vi "Radar_Wireless_2Radars.vi"(0 "VISA resource name":refnum<visa-resource-name>="COM1", 1 "baud rate":u32=9600, 4 "data bits":u16=8 min=5 max=8 step=1, 5 "parity":u16(ring) items=["None", "Odd", "Even", "Mark", "Space"], 7 "stop bits":u16(ring)=10 items=["1.0"=10, "1.5"=15, "2.0"=20], 9 "XON Character":u8=17 format="%.0x", 14 "XOFF Character":u8=19 format="%.0x", 15 "timeout (ms)":u32=10000, 21 "End read on termination character?":bool=TRUE, 24 "termination char\n(0xA = '\\n' = LF)":u8=10 format="%.0x", 25 "Input\nbuffer size":u32=4096) -> ()   [LabVIEW 2010]
doc: "The Advanced Serial Read and Write example performs a Serial Port Read, a Serial Port Write, or a combination of these actions while setting some advanced serial features like buffer size, termination characters, and XON/XOFF flow control. The user selects the actions (read or write) on the front panel. If both are selected, the VI will write the data first, read the data and then close the VISA session that is opened to the port. \n\nThe parameters set for the serial port must match the parameters of the connected instrument or device. In this example, the bytes to read parameter specifies the number of bytes that the serial port reads. If there were more bytes at the port than the number specified in bytes to read, those bytes would not be read. Also, if you specify to read more bytes than the number of bytes actually read, you might receive a timeout error message.\n\nINSTRUCTIONS:\n1) Select the serial resource and configuration parameters (baud rate, data bits, parity, stop bits, flow control).\n2) Termination character can be enabled and set. Also, set the required input buffer size prior to running the example.\n3) Select the operations to be performed. \n4) Connect the serial port to your device. If no device is available, perform a loopback test by doing one of the following. Short pins 2 and 3 on a RS-232 cable or short pin 4 to pin 8 and pin 5 to pin 9 on a RS-485/422 cable. \n5) Run the VI to see the data read. (The \"read string\" will match the \"string to write\" if a loopback test was performed.)\n\nThis example exposes several advanced features that you may need for your application. Not all applications need all the features shown in this example. The input buffer size is likely an important setting that you want to control in your application. This example expands upon the flow control option for XON and XOFF, allowing the user to choose those control characters. The timeout parameter has been brought to the front panel so a user can specify the time period the VISA Read will wait for the number of bytes to read before timing out. Also, the user has several controls for the termination character, which is discussed later.\n\nNote that you can press the write and read buttons and change the bytes to read parameters on the fly, while the example is running. However, you must stop the example to change the other configuration parameters after the example has started running, and then run again.\n\nSet the I/O buffer size slightly higher the amount of data you expect to receive. This is very important for applications that don't use flow control, as you may lose characters if the receive buffer overflows.\n\nSetting the timeout period ensures that the operation returns with a timeout error if the operation cannot be performed in the specified time period. \n\nSome devices require a termination character in order to identify the end of command strings. Some devices send a termination character to signify the end of data to be read. \n\nThis example shows how you can end the Read operation once a termination character is detected in the buffer and/or append a termination character at the end of the Write data. To enable the Read to end on a termination character, use the VISA Configure Serial Port or use the VISA Properties Serial End Mode for Reads, Termination Character Enable, and Termination Character. To end the Write with a termination character, use the VISA Properties Serial End Mode for Writes, the Send End Enable, and Termination Character. In this example, the same termination character is used for both the Read and the Write. You can specify two different characters for your application, if desired.\n\nYour application may require specific characters for the XON/XOFF Flow Control. You can specify these characters with the VISA Properties Flow Control XOFF Character and Flow Control XON Character. Note that if the standard XON and XOFF characters are used, then decimal 17 and 19 are unavailable for data values. Remember that using flow control and setting an adequate buffer size allow you to prevent buffer overflows."
uses:
  <vilib>/Instr/_visa.llb/VISA Configure Serial Port (Instr).vi
panel:
  out "I/Q channels 2":dynamicdata(graph)
  in  "Save Data":bool
  out "I/Q  Channels 1":dynamicdata(graph)
  in  "t0":timestamp=timestamp(3198752888.296 s since 1904-01-01)
  in  "FFT":i32=256
  in  "stop":bool
  in  "flow control":u16(ring) items=["None"=0, "XON/XOFF"=1, "RTS/CTS"=2, "DTR/DSR"=4]
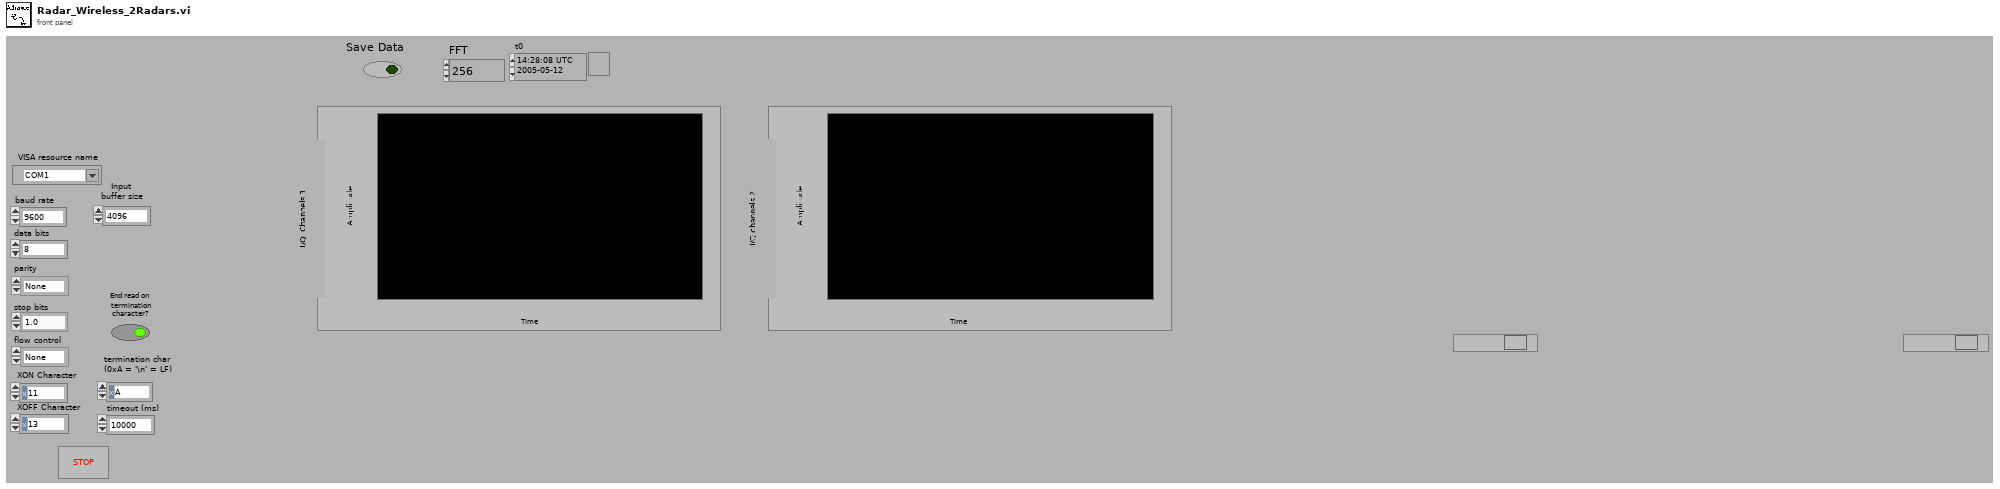
[diagram p1: front panel]
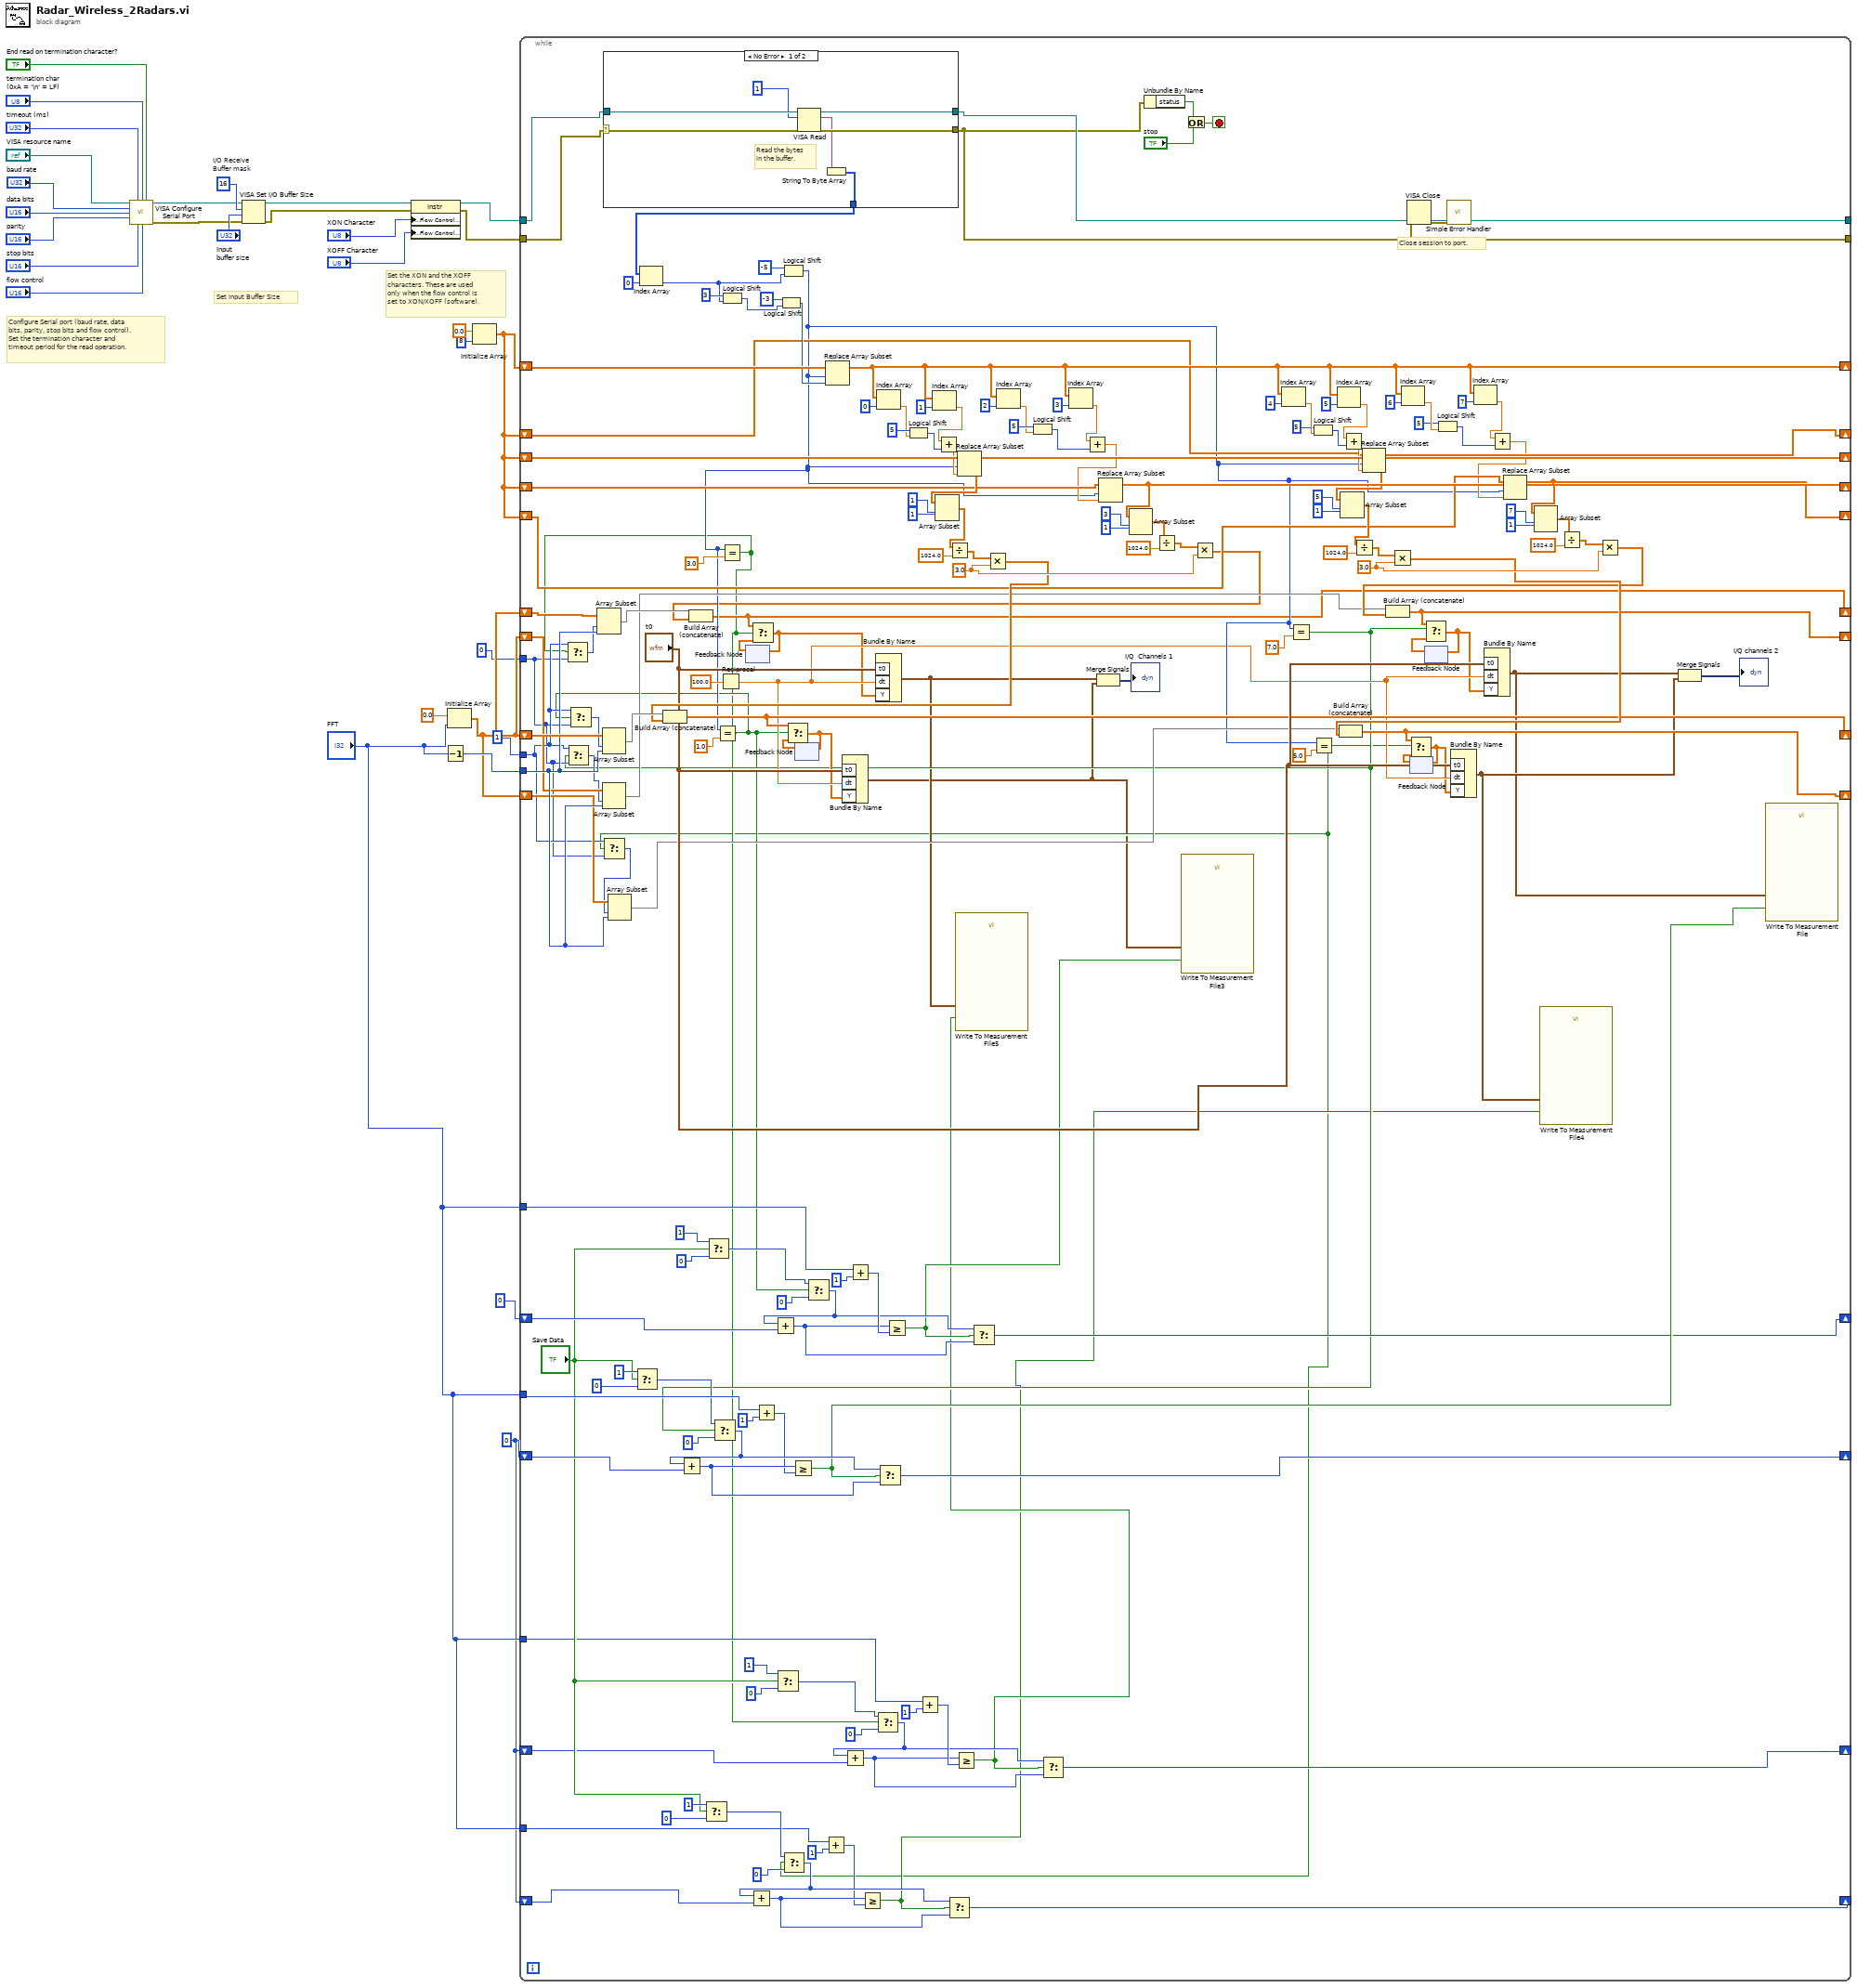
[diagram p0: block diagram]
diagram:
  w1 = 0
  w26 = u16 16  # I/O Receive Buffer mask
  # "Set the XON and the XOFF\ncharacters. These are used\nonly when the flow control is\nset to XON/XOFF (software)."
  # "Configure Serial port (baud rate, data\nbits, parity, stop bits and flow control).\nSet the termination character and\ntimeout period for the read operation."
  # "Set Input Buffer Size"
  # "Close session to port."
  n1 = call-poly "VISA Configure Serial Port"("VISA resource name"="VISA resource name", "timeout (10sec)"="timeout (ms)", "termination char\n(0xA = '\\n' = LF)"="termination char\n(0xA = '\\n' = LF)", "Enable Termination\nChar (T)"="End read on termination character?", "baud rate (9600)"="baud rate", "data bits (8)"="data bits", "parity (0:none)"="parity", "stop bits (10: 1 bit)"="stop bits", "flow control (0:none)"="flow control") -> ("VISA resource name out"=w13:refnum<visa-resource-name>, "error out"=w12:errorcluster)  [unwired: 1 in, 4 out]
  n2 = VISA Set I/O Buffer Size(VISA resource name=w13, mask (16)=w26, size (4096)="Input\nbuffer size", error in (no error)=w12) -> (VISA resource name out=w22:refnum<visa-resource-name>, error out=w21:errorcluster)
  n3 = property class="Instr"(reference=w22, error in=w21, "Serial Settings:Flow Control XON Character"="XON Character", "Serial Settings:Flow Control XOFF Character"="XOFF Character") -> (reference out=w16:refnum<visa-resource-name>, error out=w18:errorcluster)
  n4 = Decrement(x="FFT") -> (x-1=w11:i32)
  n5 = Initialize Array(0.0 ("element"), "FFT") -> (w6:dbl[])
  n6 = Initialize Array(0.0 ("element"), 8 ("dimension size")) -> (w5:dbl[])
  n7 = while {
    tunnel: w18 -> [w181]
    tunnel: w16 -> [w182]
    tunnel: [w180] -> w15
    tunnel: [w179] -> w14
    tunnel: w11 -> [w120]
    tunnel: 1 ("index") -> [w89]
    shift-right: [w103] -> _
    shift-left: w6 -> [w121]
    shift-right: [w125] -> _
    shift-left: w5 -> [w196]
    shift-right: [w93] -> _
    shift-left: w6 -> [w95]
    shift-right: [w171] -> _
    shift-left: w5 -> [w173]
    shift-right: [w164] -> _
    shift-left: w5 -> [w167]
    shift-right: [w157] -> _
    shift-left: w1 -> [w160]
    tunnel: "FFT" -> [w154]
    shift-right: [w107] -> _
    shift-left: w6 -> [w118]
    shift-right: [w100] -> _
    shift-left: w6 -> [w116]
    shift-right: [w114] -> _
    shift-left: w5 -> [w115]
    shift-right: [w112] -> _
    shift-left: w5 -> [w113]
    tunnel: 0 ("index") -> [w88]
    shift-right: [w73] -> _
    shift-left: 0 -> [w74]
    tunnel: "FFT" -> [w72]
    tunnel: "FFT" -> [w42]
    tunnel: "FFT" -> [w41]
    shift-right: [w40] -> _
    shift-left: w1 -> [w44]
    shift-right: [w43] -> _
    shift-left: w1 -> [w39]
    stop <- w205 stop-if-true
    w149 = 3.0 ("y")
    (unwired) 0
    w162 = 3.0 ("y")
    n8 = case "Read bytes from port." shown="No Error" w181 {
      selector: w181 -> [w210 w215]
      tunnel: [w212 w215] -> w179
      tunnel: [w213 w216] -> w180
      tunnel: w182 -> [w211 w216]
      tunnel: [w208 u8[] [] ("unsigned byte array")] -> w178
      frame No Error {
        # "Read the bytes\nin the buffer."
        n9 = VISA Read(VISA resource name=w211, byte count=u32 1, error in (no error)=w210) -> (VISA resource name out=w213:refnum<visa-resource-name>, read buffer=w209:string, error out=w212:errorcluster)  [unwired: 1 out]
        n10 = String To Byte Array(string=w209) -> (unsigned byte array=w208:u8[])
      }
      frame Error {
        # "Error occurred \nreading Bytes at \nSerial Port"
      }
    }
    n11 = Select(t=1, s="Save Data", f=0) -> (s? t:f=w71:i32)
    n12 = Index Array(array=w178, index=0) -> (element=w199:u8)
    n13 = Select(t=1, s="Save Data", f=0) -> (s? t:f=w50:i32)
    n14 = Select(t=1, s="Save Data", f=0) -> (s? t:f=w76:i32)
    n15 = Reciprocal(x=100.0 ("y")) -> (1/x=w97:dbl)
    n16 = Logical Shift(y=i8 3, x=w199) -> (x << y=w198:u8)
    n17 = feedback #1() -> (w94:dbl[])  [unwired: 1 out]
    n18 = Add(x=w154, y=1) -> (x+y=w155:i32)
    n19 = Select(t=1, s="Save Data", f=0) -> (s? t:f=w52:i32)
    n20 = Logical Shift(y=i8 -3, x=w198) -> (x << y=w195:u8)
    n21 = Logical Shift(y=i8 -5, x=w199) -> (x << y=w98:u8)
    n22 = Equal?(x=w98, y=1.0) -> (x = y?=w67:bool)
    n23 = Select(t=w89, s=w67, f=w88) -> (s? t:f=w91:i32)
    n24 = Array Subset(array=w121, index=w91, length=w120) -> (w203:dbl[])
    n25 = Equal?(x=w98, y=3.0) -> (x = y?=w38:bool)
    n26 = Select(t=w89, s=w38, f=w88) -> (s? t:f=w92:i32)
    n27 = Array Subset(array=w95, index=w92, length=w120) -> (w122:dbl[])
    n28 = feedback #2() -> (w104:dbl[])  [unwired: 1 out]
    n29 = Select(t=w76, s=w67, f=0) -> (s? t:f=w75:i32)
    n30 = Add(x=w75, y=w74) -> (x+y=w80:i32)
    n31 = Add(x=w41, y=1) -> (x+y=w59:i32)
    n32 = Replace Array Subset(array=w196, new element=w195, index=w98) -> (w125:dbl[])
    n33 = Add(x=w72, y=1) -> (x+y=w82:i32)
    n34 = Select(t=w52, s=w38, f=0) -> (s? t:f=w51:i32)
    n35 = Add(x=w51, y=w44) -> (x+y=w56:i32)
    n36 = Index Array(array=w125, index=0) -> (element=w189:dbl)
    n37 = Greater Or Equal?(x=w80, y=w82) -> (x >= y?=w64:bool)
    n38 = Logical Shift(y=i16 5, x=w189) -> (x << y=w185:u32)
    n39 = Add(x=w42, y=1) -> (x+y=w58:i32)
    n40 = Index Array(array=w125, index=1) -> (element=w186:dbl)
    n41 = Add(x=w186, y=w185) -> (x+y=w172:dbl)
    n42 = Greater Or Equal?(x=w56, y=w58) -> (x >= y?=w46:bool)
    n43 = Replace Array Subset(array=w173, new element=w172, index=w98) -> (w171:dbl[])
    n44 = Array Subset(array=w171, index=1, length=1) -> (w168:dbl[])
    n45 = Divide(x=w168, y=1024.0) -> (x/y=w176:dbl[])
    n46 = Select(t=w75, s=w64, f=w80) -> (s? t:f=w73:i32)
    n47 = Multiply(x=w176, y=w162) -> (x*y=w153:dbl[])
    n48 = Build Array (concatenate)(w203, w153) -> (w103:dbl[])
    n49 = Select(t=w103, s=w67, f=w104) -> (s? t:f=w83:dbl[])
    n50 = feedback-in #2(w83) -> ()
    n51 = Bundle By Name("t0"="t0", "dt"=w97, "Y"=w83) -> (w36:waveform(dbl))  [unwired: 1 out]
    n52 = Index Array(array=w125, index=2) -> (element=w187:dbl)
    n53 = Logical Shift(y=i16 5, x=w187) -> (x << y=w183:u32)
    n54 = Select(t=w51, s=w46, f=w56) -> (s? t:f=w40:i32)
    n55 = Index Array(array=w125, index=3) -> (element=w184:dbl)
    n56 = Add(x=w184, y=w183) -> (x+y=w111:dbl)
    n57 = Replace Array Subset(array=w167, new element=w111, index=w98) -> (w164:dbl[])
    n58 = Array Subset(array=w164, index=3, length=1) -> (w163:dbl[])
    n59 = Unbundle By Name(w179) -> ("status"=w206:bool)
    n60 = Divide(x=w163, y=1024.0) -> (x/y=w174:dbl[])
    n61 = call "Write To Measurement File3"("Signals"=w36, "Enable"=w64) -> ()  [unwired: 15 in, 3 out]
    n62 = Or(x=w206, y="stop") -> (x .or. y?=w205:bool)
    n63 = Multiply(x=w174, y=w162) -> (x*y=w96:dbl[])
    n64 = Build Array (concatenate)(w122, w96) -> (w93:dbl[])
    n65 = Select(t=w93, s=w38, f=w94) -> (s? t:f=w84:dbl[])
    n66 = feedback-in #1(w84) -> ()
    n67 = Bundle By Name("t0"="t0", "dt"=w97, "Y"=w84) -> (w65:waveform(dbl))  [unwired: 1 out]
    n68 = call "Write To Measurement File5"("Signals"=w65, "Enable"=w46) -> ()  [unwired: 15 in, 3 out]
    n69 = Merge Signals(w65, w36) -> (→"I/Q  Channels 1":dynamicdata)
    n70 = Index Array(array=w125, index=4) -> (element=w131:dbl)
    n71 = Equal?(x=w98, y=7.0) -> (x = y?=w68:bool)
    n72 = Select(t=w89, s=w68, f=w88) -> (s? t:f=w90:i32)
    n73 = Array Subset(array=w118, index=w90, length=w120) -> (w119:dbl[])
    n74 = Select(t=w71, s=w68, f=0) -> (s? t:f=w159:i32)
    n75 = Add(x=w159, y=w160) -> (x+y=w158:i32)
    n76 = Greater Or Equal?(x=w158, y=w155) -> (x >= y?=w151:bool)
    n77 = Select(t=w159, s=w151, f=w158) -> (s? t:f=w157:i32)
    n78 = Logical Shift(y=i16 5, x=w131) -> (x << y=w135:u32)
    n79 = Equal?(x=w98, y=5.0) -> (x = y?=w37:bool)
    n80 = Select(t=w89, s=w37, f=w88) -> (s? t:f=w87:i32)
    n81 = Array Subset(array=w116, index=w87, length=w120) -> (w117:dbl[])
    n82 = Select(t=w50, s=w37, f=0) -> (s? t:f=w62:i32)
    n83 = Add(x=w62, y=w39) -> (x+y=w61:i32)
    n84 = Greater Or Equal?(x=w61, y=w59) -> (x >= y?=w45:bool)
    n85 = Select(t=w62, s=w45, f=w61) -> (s? t:f=w43:i32)
    n86 = Index Array(array=w125, index=5) -> (element=w134:dbl)
    n87 = Add(x=w134, y=w135) -> (x+y=w142:dbl)
    n88 = Replace Array Subset(array=w113, new element=w142, index=w98) -> (w112:dbl[])
    n89 = Array Subset(array=w112, index=5, length=1) -> (w145:dbl[])
    n90 = Divide(x=w145, y=1024.0) -> (x/y=w139:dbl[])
    n91 = Multiply(x=w139, y=w149) -> (x*y=w124:dbl[])
    n92 = Build Array (concatenate)(w117, w124) -> (w100:dbl[])
    n93 = Index Array(array=w125, index=6) -> (element=w133:dbl)
    n94 = feedback #3() -> (w101:dbl[])  [unwired: 1 out]
    n95 = Select(t=w100, s=w37, f=w101) -> (s? t:f=w85:dbl[])
    n96 = feedback-in #3(w85) -> ()
    n97 = feedback #4() -> (w106:dbl[])  [unwired: 1 out]
    n98 = Logical Shift(y=i16 5, x=w133) -> (x << y=w137:u32)
    n99 = Bundle By Name("t0"="t0", "dt"=w97, "Y"=w85) -> (w35:waveform(dbl))  [unwired: 1 out]
    n100 = Index Array(array=w125, index=7) -> (element=w136:dbl)
    n101 = Add(x=w136, y=w137) -> (x+y=w110:dbl)
    n102 = Replace Array Subset(array=w115, new element=w110, index=w98) -> (w114:dbl[])
    n103 = Array Subset(array=w114, index=7, length=1) -> (w148:dbl[])
    n104 = call "Write To Measurement File4"("Signals"=w35, "Enable"=w45) -> ()  [unwired: 5 in, 13 out]
    n105 = Divide(x=w148, y=1024.0) -> (x/y=w141:dbl[])
    n106 = Multiply(x=w141, y=w149) -> (x*y=w123:dbl[])
    n107 = Build Array (concatenate)(w119, w123) -> (w107:dbl[])
    n108 = Select(t=w107, s=w68, f=w106) -> (s? t:f=w86:dbl[])
    n109 = feedback-in #4(w86) -> ()
    n110 = Bundle By Name("t0"="t0", "dt"=w97, "Y"=w86) -> (w34:waveform(dbl))  [unwired: 1 out]
    n111 = Merge Signals(w34, w35) -> (→"I/Q channels 2":dynamicdata)
    n112 = call "Write To Measurement File"("Signals"=w34, "Enable"=w151) -> ()  [unwired: 5 in, 13 out]
  }
  n113 = VISA Close(VISA resource name=w15, error in (no error)=w14) -> (error out=w31:errorcluster)
  n114 = call <vilib>:"Simple Error Handler.vi"("error in (no error)"=w31) -> ()  [unwired: 1 in, 8 out]
